vi "CH_LM App RecallSetup.vi"(2 "error in (no error)":errorcluster, 3 "Meter Index":i32) -> (0 "error out":errorcluster)   [LabVIEW 2012, in "CH_LM App.lvlib"]
doc: "This VI queries for setup configurations on the LabMax meter.\nYou can recall or delete the selected setup or save the current."
uses:
  CH_LM App.lvlib
  CH_LM.lvlib
  Instance           2 29Saved   CH_LM App RecallSetup .vi
  Instance           1 29Saved   CH_LM App RecallSetup .vi
panel:
  in  "Delete":bool
  in  "Save":bool
  in  "Cancel Button":bool
  in  "OK Button":bool
  in  "Setup Configurations":i32(listbox)
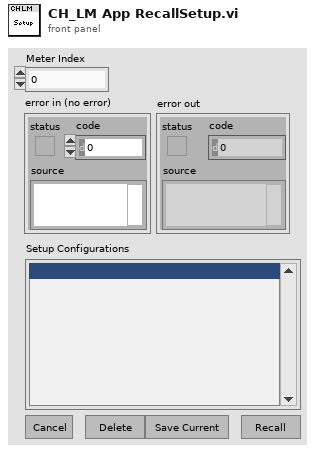
[diagram p1: front panel]
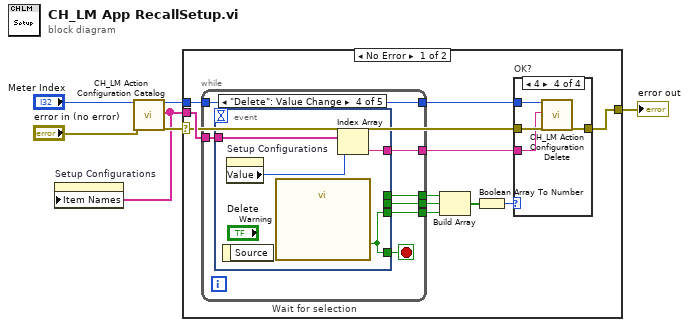
[diagram p0: block diagram]
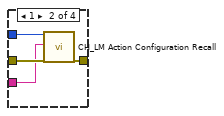
[diagram p3: hidden frame]
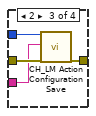
[diagram p4: hidden frame]
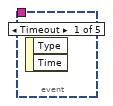
[diagram p5: hidden frame]
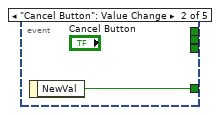
[diagram p6: hidden frame]
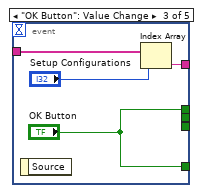
[diagram p7: hidden frame]
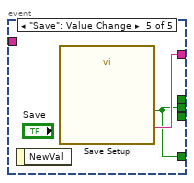
[diagram p8: hidden frame]
diagram:
  n1 = call "CH_LM Action Configuration Catalog.vi"("Meter Index"="Meter Index", "error in (no error)"="error in (no error)") -> ("Meter Index"=w6:i32, "Configuration Catalog"=w2:string[], "error out"=w3:errorcluster)  [unwired: 15 out]
  n2 = property on="Setup Configurations" class="LstBox (strict)"("Item Names"=w2) -> ()  [unwired: 2 in, 2 out]
  n3 = case shown="No Error" w3 {
    selector: w3 -> [w14 w49]
    tunnel: w6 -> [w16 _]
    tunnel: [w13 w49] -> w1
    tunnel: w2 -> [w17 _]
    frame No Error {
      n4 = while "Wait for selection" {
        tunnel: [w36] -> w11
        tunnel: w17 -> [w35]
        tunnel: w16 -> [w34]
        tunnel: [w34] -> w15
        tunnel: [w33] -> w12
        tunnel: [w32] -> w10
        tunnel: [w31] -> w7
        stop <- w37 stop-if-true
        n5 = event shown="[3] \"Delete\": Value Change" {
          selector: _ -> [_ _ _ _ _]
          dyn-events: _ -> [_ _ _ _ _]
          timeout: _ -> [_ _ _ _ _]
          tunnel: [_ w38 "OK Button" w43 w47] -> w37
          tunnel: [_ _ _ _ w47] -> w36
          tunnel: w35 -> [_ _ w42 w46 _]
          tunnel: [_ _ w40 w45 w48] -> w33
          tunnel: [_ _ "OK Button" _ _] -> w32
          tunnel: [_ _ _ w43 _] -> w31
          event Timeout {
            n6 = event-data() -> ()  [unwired: 3 out]
          }
          event "Cancel Button": Value Change {
            n7 = event-data() -> ("NewVal"=w38:bool)  [unwired: 1 out]
          }
          event "OK Button": Value Change {
            n8 = event-data() -> ()  [unwired: 2 out]
            n9 = Index Array(array=w42, index="Setup Configurations") -> (element=w40:string)
          }
          event "Delete": Value Change {
            n10 = event-data() -> ()  [unwired: 2 out]
            n11 = property on="Setup Configurations" class="LstBox (strict)"() -> ("Value"=w44:i32)  [unwired: 2 in, 2 out]
            n12 = call "Warning"() -> ("OK"=w43:bool)  [unwired: 2 in, 17 out]
            n13 = Index Array(array=w46, index=w44) -> (element=w45:string)
          }
          event "Save": Value Change {
            n14 = event-data() -> ()  [unwired: 2 out]
            n15 = call "Save Setup"() -> ("Setup Name"=w48:string, "OK"=w47:bool)  [unwired: 2 in, 16 out]
          }
        }
      }
      n16 = Build Array(w10, w11, w7) -> (w9:bool[])
      n17 = Boolean Array To Number(Boolean array=w9) -> (number=w8:u32)
      n18 = case "OK?" shown="4" w8 {
        tunnel: w15 -> [_ w22 w26 w29]
        tunnel: w14 -> [w18 w21 w25 w30]
        tunnel: [w18 w20 w24 w28] -> w13
        tunnel: w12 -> [_ w19 w23 w27]
        frame 0, Default {
        }
        frame 1 {
          n19 = call "CH_LM Action Configuration Recall.vi"("Meter Index"=w22, "Configuration File Name (\"\")"=w19, "error in (no error)"=w21) -> ("error out"=w20:errorcluster)  [unwired: 16 out]
        }
        frame 2 {
          n20 = call "CH_LM Action Configuration Save.vi"("Meter Index"=w26, "Configuration File Name (\"\")"=w23, "error in (no error)"=w25) -> ("error out"=w24:errorcluster)  [unwired: 16 out]
        }
        frame 4 {
          n21 = call "CH_LM Action Configuration Delete.vi"("Meter Index"=w29, "Configuration File Name (\"\")"=w27, "error in (no error)"=w30) -> ("error out"=w28:errorcluster)  [unwired: 16 out]
        }
      }
    }
    frame Error {
    }
  }
  "error out" <- w1
